vi "Write Key (Raw).vi"(7 "Section Name":string, 8 "error in (no error)":errorcluster, 9 "Content":string, 10 "Key Name":string, 11 "Config in":T1) -> (0 "error out":errorcluster, 2 "Key Replaced?":bool, 3 "Config out":T1)   [LabVIEW 2022 SP3, in "LabVIEW-Config.lvlib"]
uses:
  LabVIEW-Config.lvlib
  Config.ctl
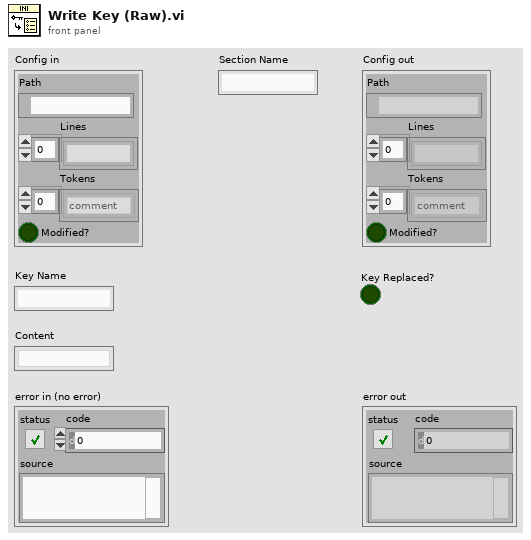
[diagram p1: front panel]
types:
  T1 = typedef "LabVIEW-Config.lvlib/Config.ctl" = cluster{"Path":path, "Lines":string[], "Tokens":enum8{"comment", "section", "key"}[], "Modified?":bool}
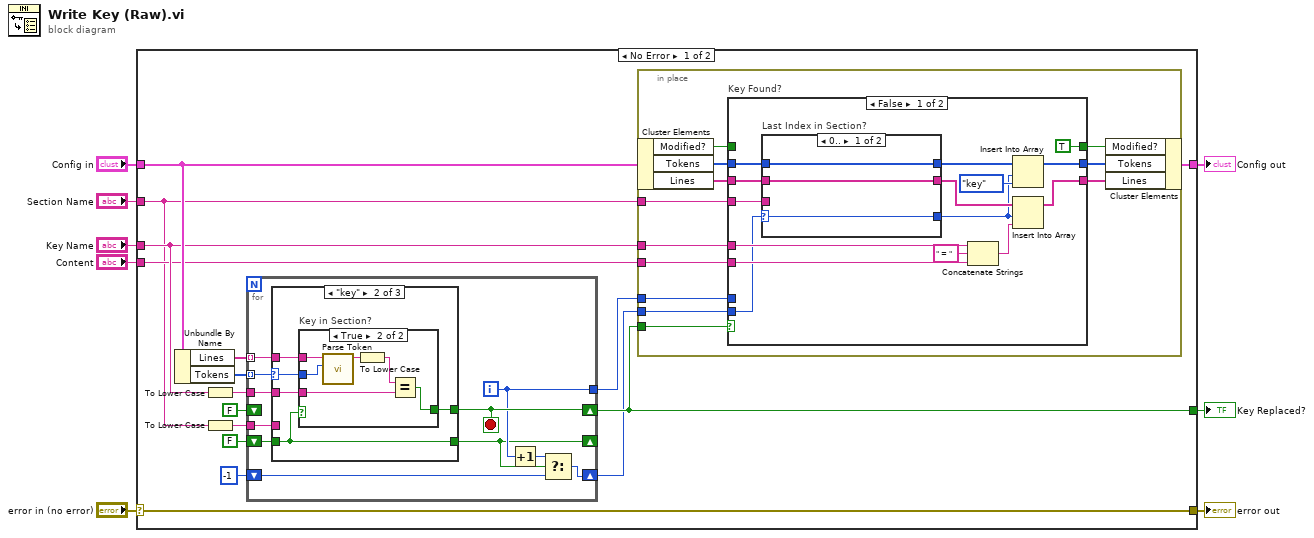
[diagram p0: block diagram]
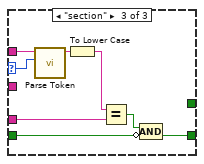
[diagram p4: hidden frame]
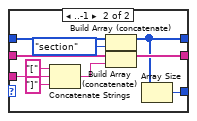
[diagram p5: hidden frame]
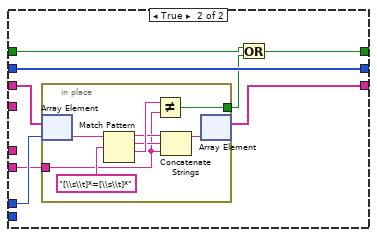
[diagram p6: hidden frame]
diagram:
  n1 = case shown="No Error" "error in (no error)" {
    selector: "error in (no error)" -> [w22 w113]
    tunnel: "Config in" -> [w15 w112]
    tunnel: [w22 w113] -> w7
    tunnel: [w9 w112] -> w5
    tunnel: "Section Name" -> [w10 _]
    tunnel: [w17 _] -> w3
    tunnel: "Key Name" -> [w12 _]
    tunnel: "Content" -> [w11 _]
    frame No Error {
      n2 = Unbundle By Name(w15) -> ("Lines"=w23:string[], "Tokens"=w24:enum8{"comment", "section", "key"}[])
      n3 = To Lower Case(string=w12) -> (all lower case string=w18:string)
      n4 = To Lower Case(string=w10) -> (all lower case string=w21:string)
      n5 = for {
        tunnel: w24 -> [w35] mode=indexing
        tunnel: w23 -> [w34] mode=indexing
        tunnel: w21 -> [w33]
        shift-right: [w25] -> _
        shift-left: FALSE -> [w27]
        shift-right: [w31] -> w17
        shift-left: FALSE -> [_]
        tunnel: w18 -> [w32]
        tunnel: [w30] -> w14
        shift-right: [w29] -> w13
        shift-left: -1 -> [w28]
        i -> [w30]
        stop <- w31 stop-if-true
        n6 = case shown="\"key\"" w35 {
          selector: w35 -> [_ w37 w48]
          tunnel: w34 -> [_ w41 w50]
          tunnel: w33 -> [_ _ w55]
          tunnel: [w36 w40 w51] -> w25
          tunnel: w27 -> [w36 w40 w53]
          tunnel: w32 -> [_ w39 _]
          tunnel: [_ w38 _] -> w31
          frame "comment" {
          }
          frame "key" {
            n7 = case "Key in Section?" shown="True" w40 {
              tunnel: w41 -> [_ w44]
              tunnel: w39 -> [_ w47]
              tunnel: [_ w45] -> w38
              tunnel: w37 -> [_ w43]
              frame False {
              }
              frame True {
                n8 = call "Parse Token.vi"("Token"=w43, "Line"=w44) -> ("Name"=w42:string)  [unwired: 8 in, 1 out]
                n9 = To Lower Case(string=w42) -> (all lower case string=w46:string)
                n10 = Equal?(x=w46, y=w47) -> (x = y?=w45:bool)
              }
            }
          }
          frame "section" {
            n11 = call "Parse Token.vi"("Token"=w48, "Line"=w50) -> ("Name"=w49:string)  [unwired: 8 in, 1 out]
            n12 = To Lower Case(string=w49) -> (all lower case string=w54:string)
            n13 = Equal?(x=w54, y=w55) -> (x = y?=w52:bool)
            n14 = Compound Arithmetic op=AND(w52, invert w53) -> (w51:bool)
          }
        }
        n15 = Increment(x=w30) -> (x+1=w26:i32)
        n16 = Select(t=w26, s=w25, f=w28) -> (s? t:f=w29:i32)
      }
      n17 = in-place {
        in-place-border: w17 -> [w67]
        in-place-border: w14 -> [w60]
        in-place-border: w13 -> [w59]
        in-place-border: w12 -> [w58]
        in-place-border: w11 -> [w57]
        in-place-border: w10 -> [w56]
        n18 = in-place-cluster #1(w15) -> ("Modified?"=w62:bool, "Tokens"=w66:enum8{"comment", "section", "key"}[], "Lines"=w65:string[])
        n19 = case "Key Found?" shown="False" w67 {
          tunnel: w66 -> [w81 w102]
          tunnel: w65 -> [w80 w101]
          tunnel: [w78 w102] -> w64
          tunnel: [w79 w100] -> w63
          tunnel: w62 -> [_ w96]
          tunnel: [TRUE ("Modified?") w97] -> w61
          tunnel: w59 -> [w68 _]
          tunnel: w58 -> [w77 _]
          tunnel: w57 -> [w76 w99]
          tunnel: w56 -> [w70 _]
          tunnel: w60 -> [_ w103]
          frame False {
            n20 = case "Last Index in Section?" shown="0.." w68 {
              selector: w68 -> [w83 _]
              tunnel: w81 -> [w85 w88]
              tunnel: w80 -> [w84 w95]
              tunnel: [w85 w86] -> w72
              tunnel: [w84 w94] -> w71
              tunnel: w70 -> [_ w92]
              tunnel: [w83 w87] -> w69
              frame 0.. {
              }
              frame ..-1 {
                n21 = Concatenate Strings("[" ("string"), w92, "]" ("string")) -> (w89:string)
                n22 = Build Array (concatenate)(w88, enum8{"comment", "section", "key"}."section" ("new element/subarray")) -> (w86:enum8{"comment", "section", "key"}[])
                n23 = Build Array (concatenate)(w95, w89) -> (w94:string[])
                n24 = Array Size(array=w86) -> (size(s)=w87:i32)
              }
            }
            n25 = Concatenate Strings(w77, " = " ("string"), w76) -> (w73:string)
            n26 = Insert Into Array(array=w72, index=w69, new element=enum8{"comment", "section", "key"}."key" ("new element/subarray")) -> (w78:enum8{"comment", "section", "key"}[])
            n27 = Insert Into Array(array=w71, index=w69, new element=w73) -> (w79:string[])
          }
          frame True {
            n28 = in-place {
              in-place-border: w99 -> [w106]
              in-place-border: [w104] -> w98
              n29 = in-place-array #2(w101, w103) -> (w110:string)
              n30 = Match Pattern(string=w110, regular expression="[\\s\\t]*=[\\s\\t]*") -> (before substring=w108:string, match substring=w107:string, after substring=w109:string)  [unwired: 1 in, 1 out]
              n31 = Not Equal?(x=w109, y=w106) -> (x != y?=w104:bool)
              n32 = Concatenate Strings(w108, w107, w106) -> (w105:string)
              n33 = in-place-array #2(w105) -> (w100:string[])  [unwired: 1 out]
            }
            n34 = Or(x=w96, y=w98) -> (x .or. y?=w97:bool)
          }
        }
        n35 = in-place-cluster #1("Modified?"=w61, "Tokens"=w64, "Lines"=w63) -> (w9:T1)
      }
    }
    frame Error {
    }
  }
  "error out" <- w7
  "Config out" <- w5
  "Key Replaced?" <- w3
